vi "RobotStates.vi"() -> ()   [LabVIEW 2018]
panel:
  in  "Climber Foot State":bool
  out "Check Limit Switch":bool
  out "Elevator Motor Failure":bool
  in  "Elevator Goal (in)":dbl
  out "End of Match":bool
  in  "Max Climb Power":dbl
  in  "Climb Sequence String":string
  in  "LimeLight Pipeline":dbl
  in  "Climb Sequence":i32
  out "Tilt Interlock Engaged":bool
  out "State_Conflict_Light":bool
  out "COM Warning":bool
  out "Elevator Moving":bool
  in  "Auto Stow Sequence":i32
  in  "Auto Stow":bool
  in  "LimeLight Cam Mode":dbl
  in  "LimeLight LED Mode":dbl
  in  "Autopilot":bool
  in  "Climb Started":bool
  out "State_Conflict":bool
  in  "Lower Pulse State":bool
  in  "Lower Valve State":bool
  in  "Upper Pulse State":bool
  in  "Climber Mantis State":bool
  in  "PTO State":bool
  in  "Spare Power":dbl
  in  "HATCH Ejection":bool
  in  "HATCH Ejection Allowed":bool
  in  "HATCH Arm":bool
  in  "Elevator Brake State":bool
  out "Compressor State":bool
  in  "Vacuum Pump Power":dbl
  in  "Drive Left Side Power":dbl
  in  "Drive Right Side Power":dbl
  in  "Elevator Power":dbl
  in  "Lower Intake Power":dbl
  in  "Upper Intake Power":dbl
  in  "CARGO Intake Allowed":bool
  out "Elevator State":string
  out "Elevator State Names":string[](array[string])
  in  "CARGO Arm":bool
  in  "Upper Valve State":bool
  in  "Shifter State":bool
  in  "Butterfly State":bool
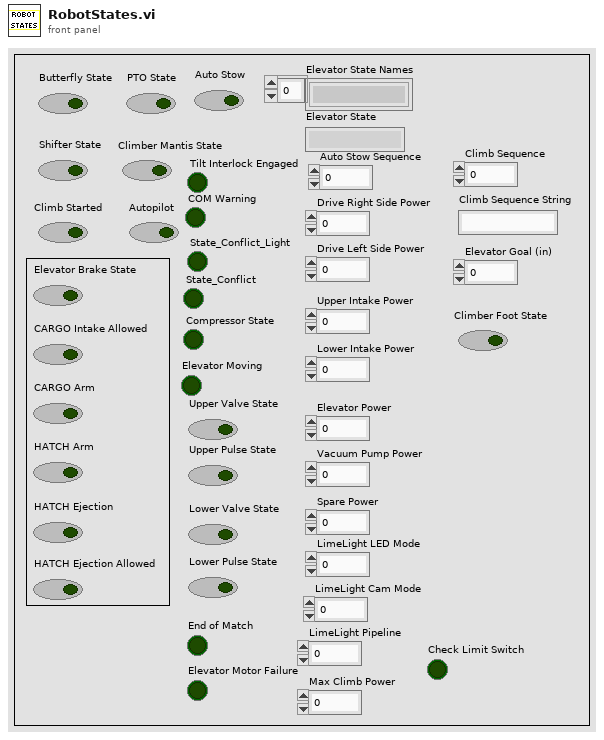
[diagram p1: front panel]
diagram:
